vi "Periodic Tasks.vi"(8 "error in":errorcluster) -> ()   [LabVIEW 2014]
doc: "This VI runs in parallel to other tasks. It can contain as many user-defined periodic loops as you need. These can carry out PID or other sorts of timed response."
uses:
  Robot Global Data.vi
panel:
  out "Slide A 2":dbl(slide) scale=0.0..60.0
  out "Slide A":dbl(slide) scale=0.0..60.0
  out "Lift B Height":dbl format="%#_13g"
  out "Lift A Height":dbl format="%#_13g"
  in  "Reset Zero Position":bool
  out "Angle":dbl(knob) scale=0.0..360.0
  in  "stop":bool
  in  "# Items to Lift":i32=1 min=0 max=4 step=1
  out "A Up":dbl
  out "A Down":dbl
  out "B Up":dbl
  out "B Down":dbl
  out "Encoder B":dbl
  out "Encoder A":dbl
  out "Rate B":dbl
  out "Rate A":dbl
  in  "Arcade Drive?":bool
  # "Adjust the Move Lift Parameters\nto  control the speed of each lift."
  # "Tank Drive Indicators"
  # "GYRO Stuff Here"
  # "This will display the current gyro angle."
  # "The items to lift control the motor gain for raising\nand lowering in different situations.  There is a zero setting\nfor moving the motors without a tote.\n\nTo change these go to the Global Variable section and change\nthe items there (make them the default settings)."
  # "This can be set while running."
  # "Analog Devices\nADW22307"
  # "Generic Gyro Wiring:\nroboRIO AI0 S (white wire) to gyro RATE\nroboRIO AI0 V (red wire) to gyro 5V\nroboRIO AI0     (black wire) to gyro GND"
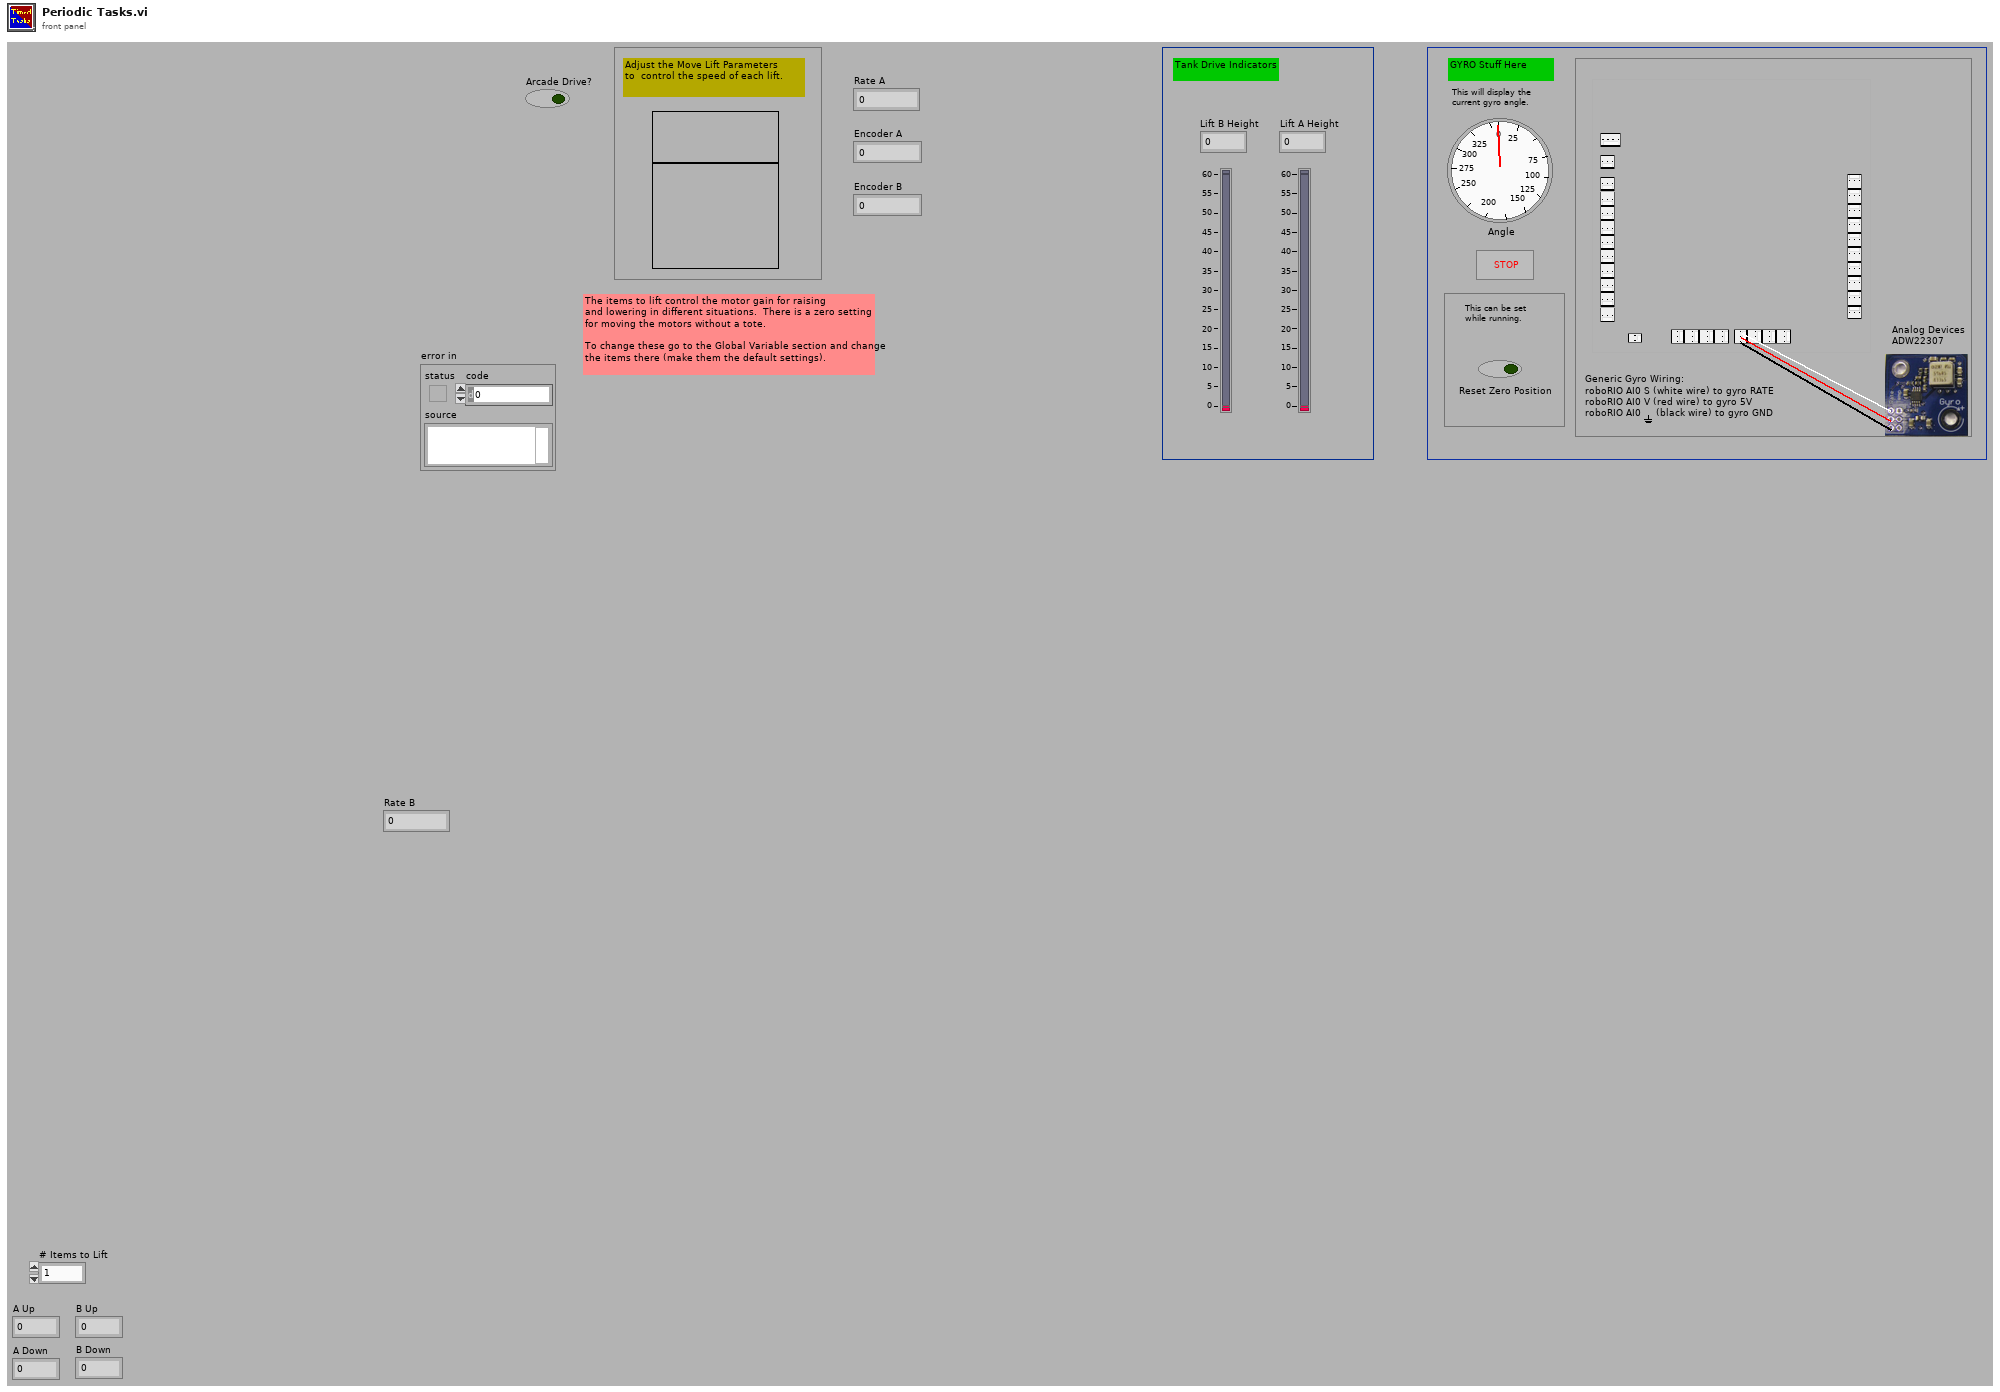
[diagram p1: front panel]
types:
  T1 = typedef "WPI_EncoderDevRef.ctl" = cluster{"DevStatus":errorcluster, "EncoderIndex":T2, "CounterIndex":T3, "DistancePerCount":dbl, "Decoding Type":T4}
  T2 = typedef "FPGA_EncoderIdx.ctl" = enum8{"Enc 0", "Enc 1", "Enc 2", "Enc 3", "Enc 4", "Enc 5", "Enc 6", "Enc 7", "Invalid"}
  T3 = typedef "FPGA_CounterCtrSystemIndex.ctl" = enum8{"Ctr 0", "Ctr 1", "Ctr 2", "Ctr 3", "Ctr 4", "Ctr 5", "Ctr 6", "Ctr 7", "Invalid"}
  T4 = typedef "WPI_EncoderType.ctl" = enum16{"1x", "2x", "4x"}
  T5 = typedef "WPI_RobotDriveDevRef.ctl" = cluster{"DevStatus":errorcluster, "Motors[]":T6[], "Square Inputs":bool, "Max Output":dbl}
  T6 = typedef "WPI_MotorControlDeviceRef.ctl" = cluster{"DeviceStatus":errorcluster, "Type":T7, "PWM":cluster{"Controller":T8, "PWM Channel":T9, "DeadBand":T10}, "CAN":cluster{"Device Number":u8, "Control Mode":T11, "Semaphore":T12, "Max Vout":dbl, "TalonSRX Control Mode":T13}, "Invert":bool, "TransformRef":T14, "InvTransformRef":T14}
  T7 = typedef "WPI_MotorControlType.ctl" = enum16{"PWM", "CAN", "CANTalonSRX"}
  T8 = typedef "FPGA_TypedefDigitalModule.ctl" = enum16{"Controller 1"}
  T9 = typedef "FPGA_DIOPWMChannel.ctl" = enum8{"PWM 0", "PWM 1", "PWM 2", "PWM 3", "PWM 4", "PWM 5", "PWM 6", "PWM 7", "PWM 8", "PWM 9", "PWM MXP 0", "PWM MXP 1", "PWM MXP 2", "PWM MXP 3", "PWM MXP 4", "PWM MXP 5", "PWM MXP 6", "PWM MXP 7", "PWM MXP 8", "PWM MXP 9", "Invalid"}
  T10 = typedef "WPI_PWMDeadband.ctl" = cluster{"Name":string, "maxPositivePwm":i32, "minPositivePwm":i32, "centerPwm":i32, "maxNegativePwm":i32, "minNegativePwm":i32, "angularRange":u16}
  T11 = typedef "WPI_CANJaguar_ControlMode.ctl" = enum8{"Percent VBus", "Current", "Speed", "Position", "Voltage"}
  T12 = typedef "Semaphore RefNum" = refnum<k1>
  T13 = typedef "WPI_CANTalonSRX_APIControlMode.ctl" = enum8{"Percent VBus", "Speed", "Position", "Slave", "Unchanged / Invalid"}
  T14 = typedef "WPI_PWMTransform_ConPane.ctl" = refnum<vi>
  T15 = typedef "WPI_JoystickDevRef.ctl" = cluster{"Device":T16}
  T16 = typedef "WPI_JoystickDeviceEnum.ctl" = enum16{"USB 0", "USB 1", "USB 2", "USB 3", "USB 4", "USB 5"}
  T17 = cluster{"Axes[0]":dbl, "Axes[1]":dbl, "Axes[2]":dbl, "Axes[3]":dbl, "Axes[4]":dbl, "Axes[5]":dbl, "Axes[6]":dbl, "Axes[7]":dbl, "Axes[8]":dbl}
  T18 = cluster{"JoystickDevRef":T15, "RobotDriveDevRef":T5}
  T19 = typedef "WPI_GyroDevRef.ctl" = cluster{"DevStatus":errorcluster, "Analog Module":T20, "Analog Channel":T21, "Offset":dbl, "Gain (VoltsPerDegree/Second)":dbl}
  T20 = typedef "FPGA_TypedefAnalogModule.ctl" = enum16{"Controller 1"}
  T21 = typedef "FPGA_AIChannel.ctl" = enum8{"AI 0", "AI 1", "AI 2", "AI 3", "AI MXP 0", "AI MXP 1", "AI MXP 2", "AI MXP 3", "Invalid"}
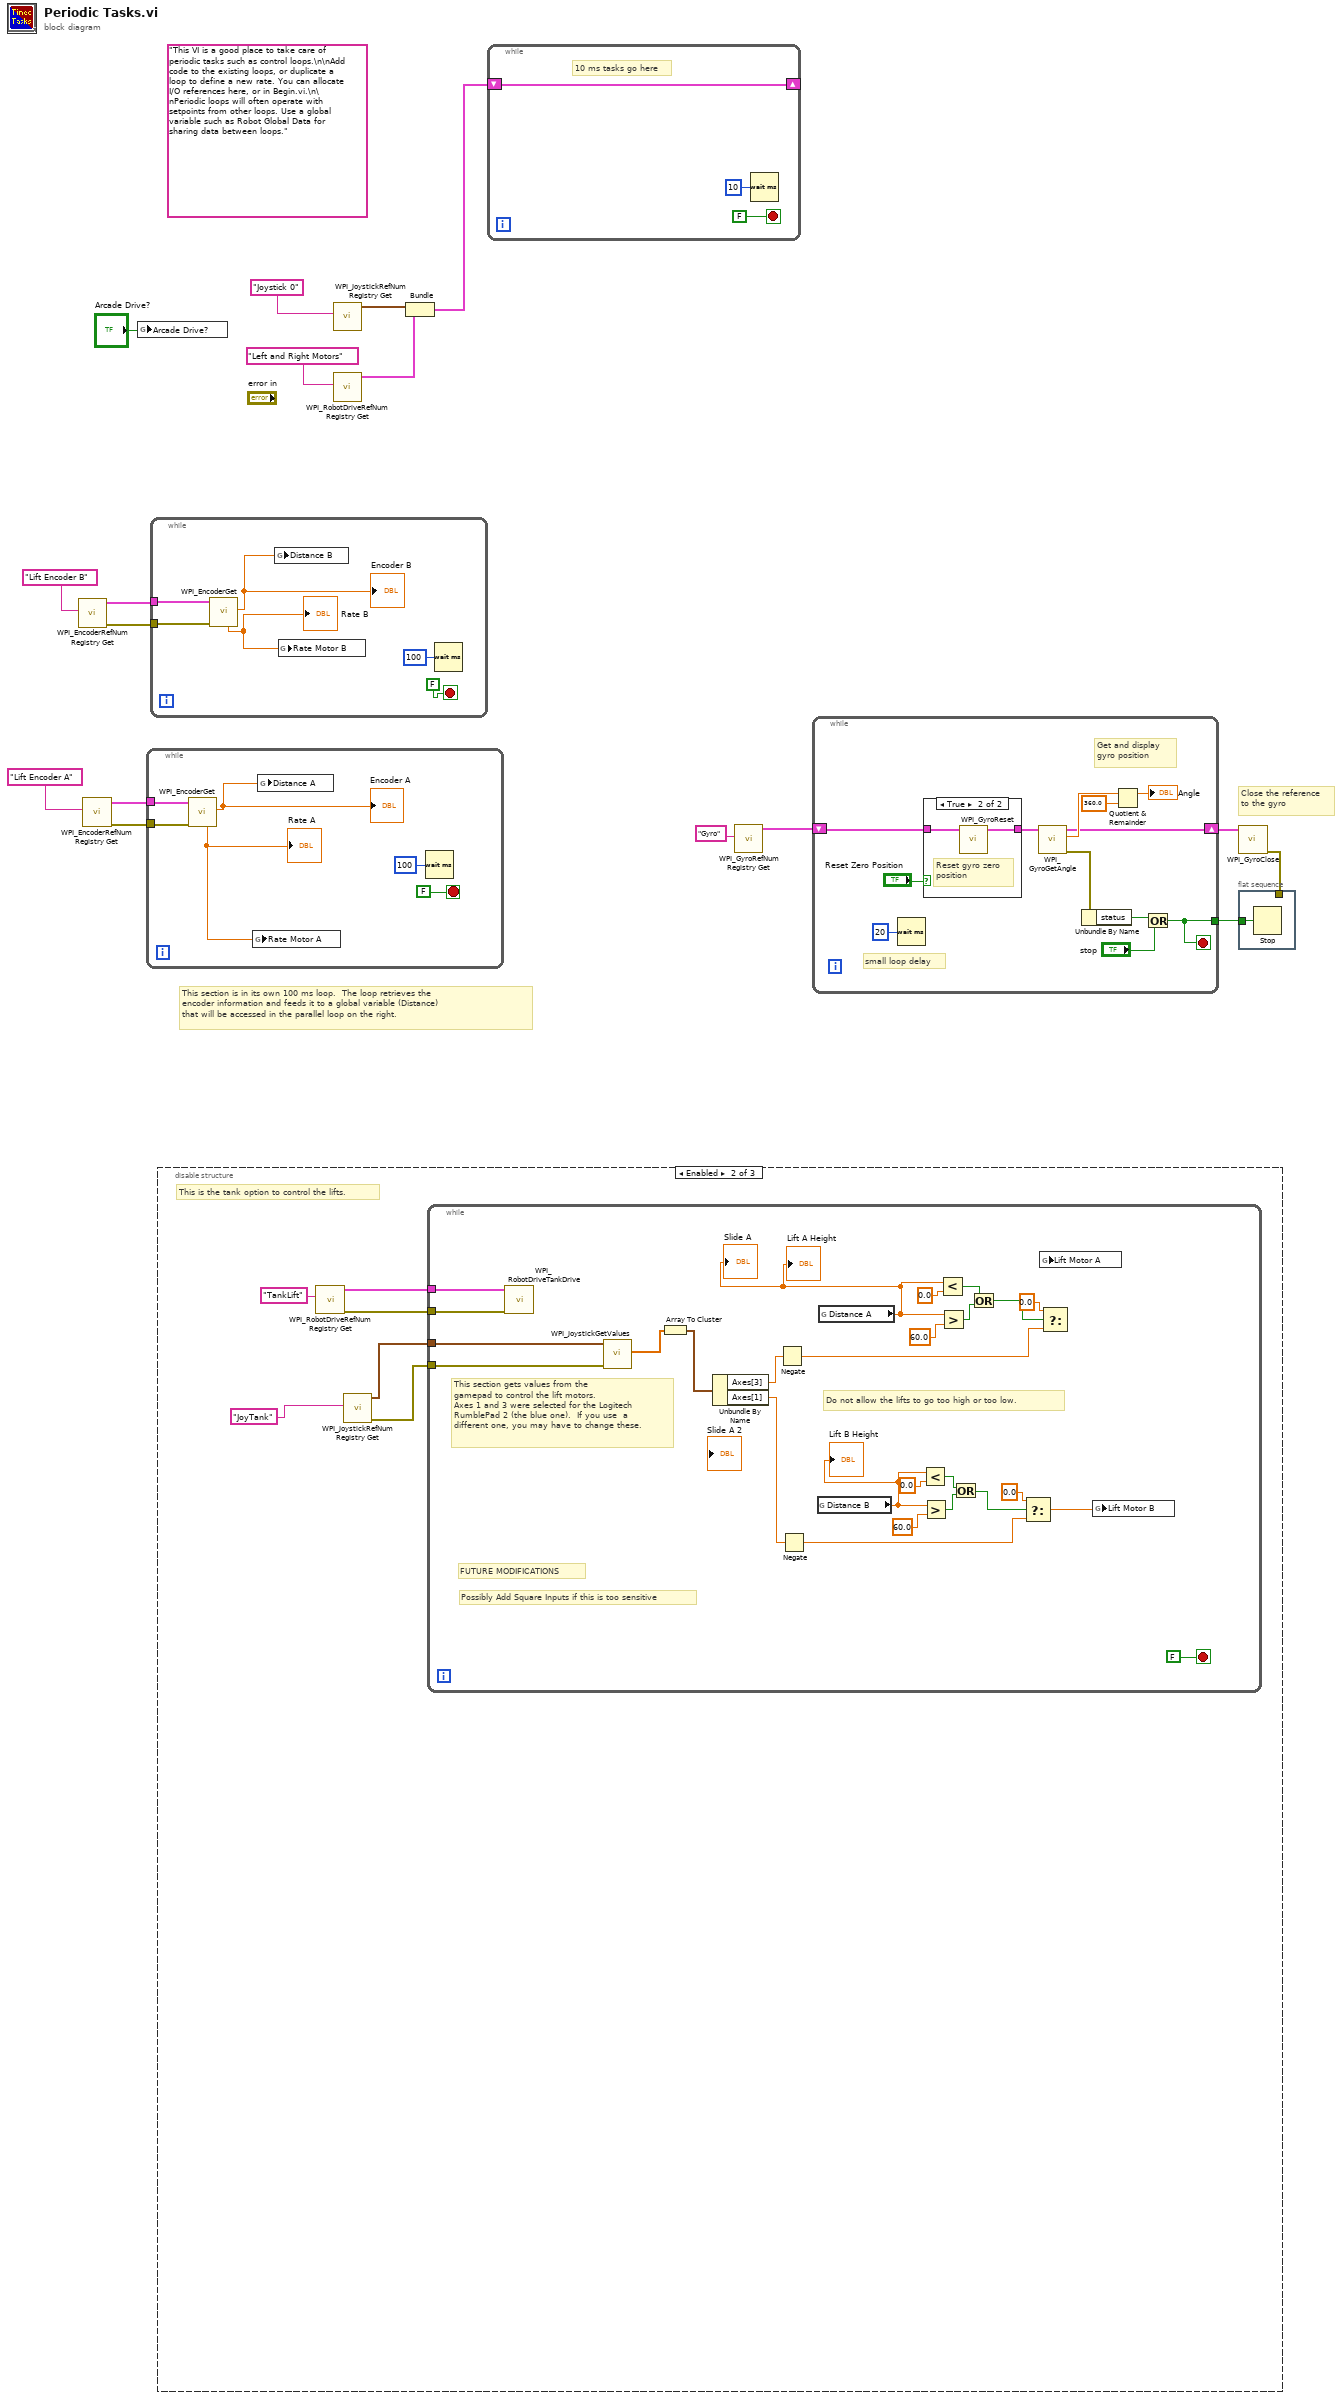
[diagram p0: block diagram]
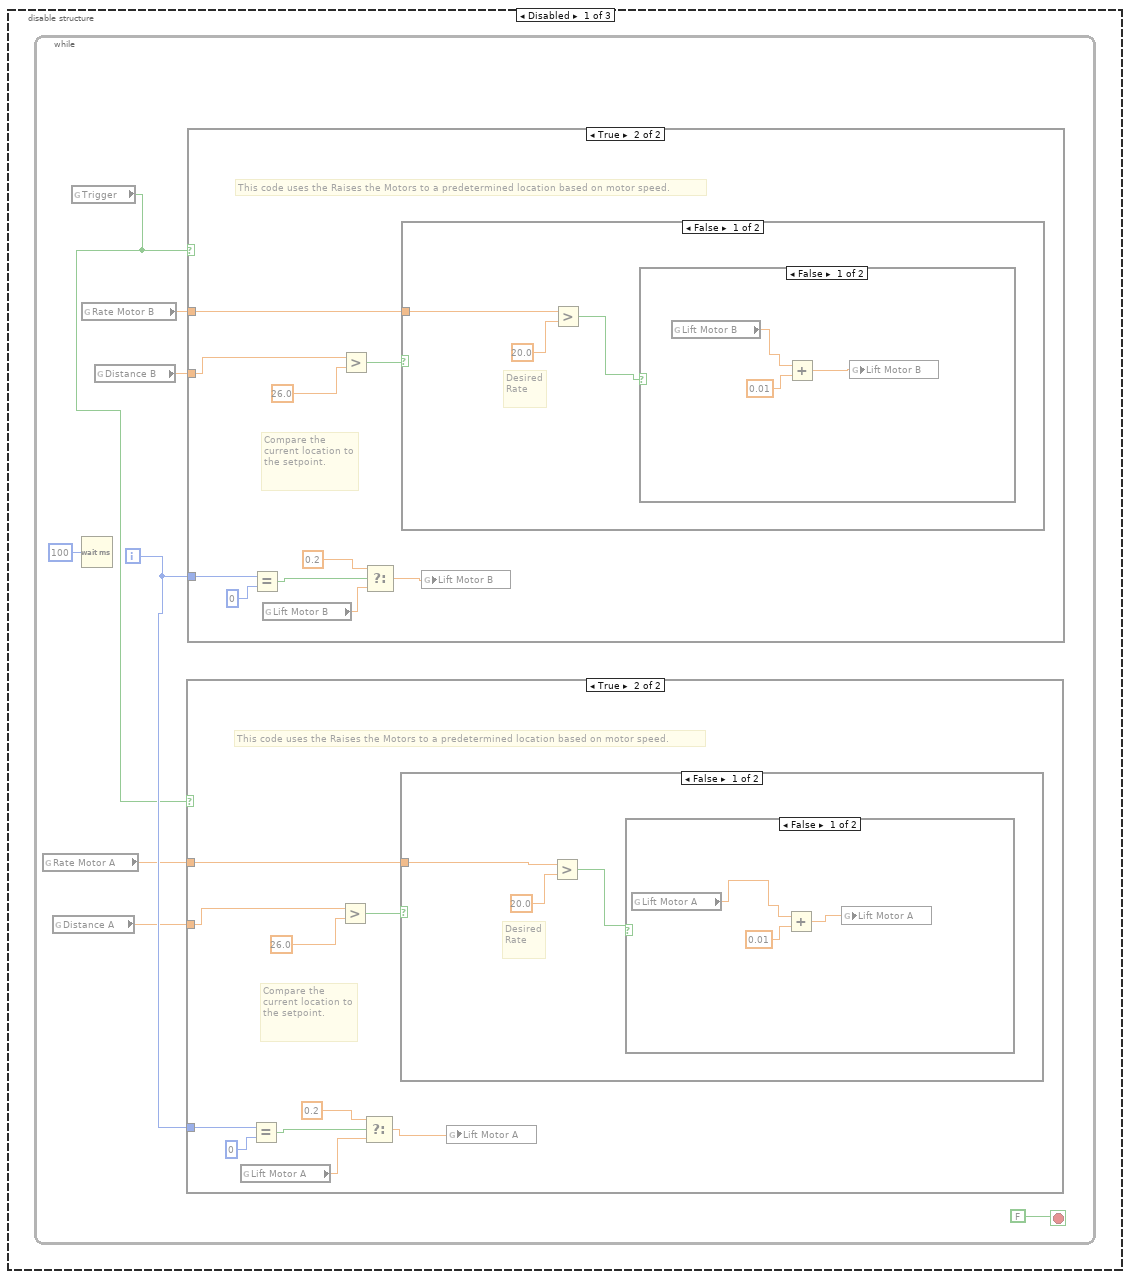
[diagram p3: hidden frame]
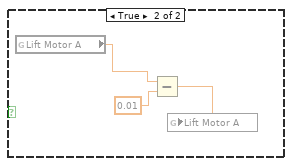
[diagram p5: hidden frame]
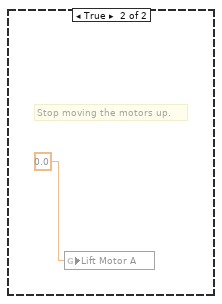
[diagram p6: hidden frame]
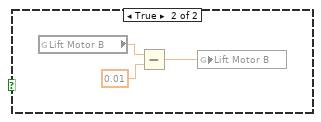
[diagram p8: hidden frame]
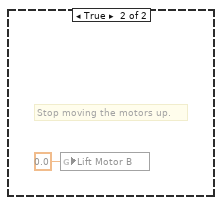
[diagram p9: hidden frame]
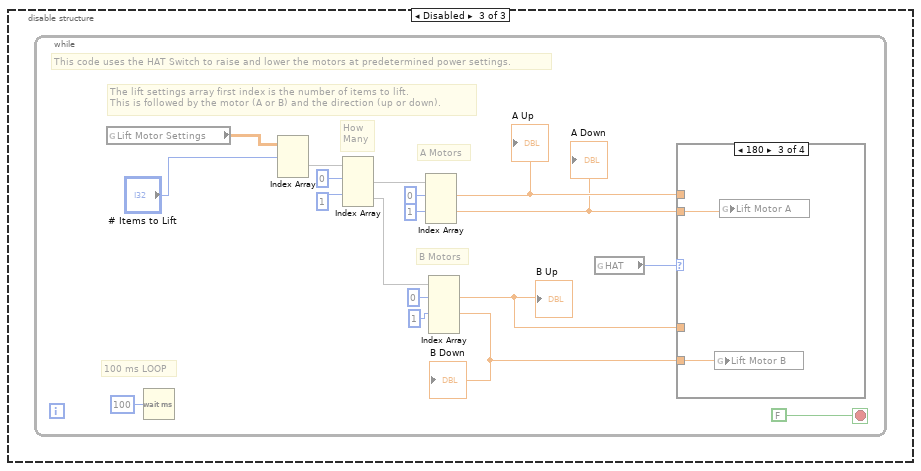
[diagram p10: hidden frame]
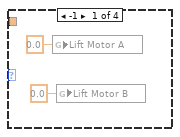
[diagram p11: hidden frame]
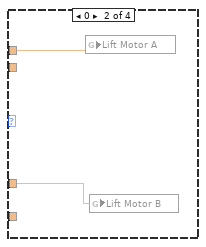
[diagram p12: hidden frame]
diagram:
  (unwired) "This VI is a good place to take care of periodic tasks such as control loops.\n\nAdd code to the existing loops, or duplicate a loop to define a new rate. You can allocate I/O references here, or in Begin.vi.\n\nPeriodic loops will often operate with setpoints from other loops. Use a global variable such as Robot Global Data for sharing data between loops."
  # "Close the reference\nto the gyro"
  # "This section is in its own 100 ms loop.  The loop retrieves the\nencoder information and feeds it to a global variable (Distance)\nthat will be accessed in the parallel loop on the right."
  n1 = call <vilib>:"WPI_EncoderRefNum Registry Get.vi"("refnum name"="Lift Encoder B") -> ("error out"=w6:errorcluster, "EncoderDevRef"=w7:T1)  [unwired: 9 in]
  n2 = call <vilib>:"WPI_EncoderRefNum Registry Get.vi"("refnum name"="Lift Encoder A") -> ("error out"=w8:errorcluster, "EncoderDevRef"=w9:T1)  [unwired: 9 in]
  n3 = global write "Robot Global Data.vi" "Arcade Drive?"("Arcade Drive?") -> ()
  n4 = while {
    tunnel: w9 -> [w21]
    tunnel: w8 -> [w20]
    stop <- FALSE stop-if-true
    n5 = call <vilib>:"WPI_EncoderGet.vi"("error in (no error)"=w20, "EncoderDevRef"=w21) -> ("Distance"=w19:dbl, "Rate"=w18:dbl)  [unwired: 4 in, 4 out]
    "Rate A" <- w18
    "Encoder A" <- w19
    n6 = global write "Robot Global Data.vi" "Rate Motor A"(w18) -> ()
    n7 = global write "Robot Global Data.vi" "Distance A"(w19) -> ()
    n8 = Wait (ms)(milliseconds to wait=u32 100) -> ()  [unwired: 1 out]
  }
  n9 = while {
    tunnel: w7 -> [w27]
    tunnel: w6 -> [w26]
    stop <- FALSE stop-if-true
    n10 = call <vilib>:"WPI_EncoderGet.vi"("error in (no error)"=w26, "EncoderDevRef"=w27) -> ("Distance"=w29:dbl, "Rate"=w28:dbl)  [unwired: 4 in, 4 out]
    "Rate B" <- w28
    "Encoder B" <- w29
    n11 = global write "Robot Global Data.vi" "Distance B"(w29) -> ()
    n12 = global write "Robot Global Data.vi" "Rate Motor B"(w28) -> ()
    n13 = Wait (ms)(milliseconds to wait=u32 100) -> ()  [unwired: 1 out]
  }
  n14 = disable-structure shown="Enabled" {
    frame Disabled {
      n15 = while {
        i -> [w33]
        stop <- FALSE stop-if-true
        n16 = global read "Robot Global Data.vi" "Rate Motor A"() -> (w31:dbl)
        n17 = global read "Robot Global Data.vi" "Distance A"() -> (w30:dbl)
        n18 = global read "Robot Global Data.vi" "Trigger"() -> (w32:bool)
        n19 = global read "Robot Global Data.vi" "Rate Motor B"() -> (w34:dbl)
        n20 = Wait (ms)(milliseconds to wait=u32 100) -> ()  [unwired: 1 out]
        n21 = global read "Robot Global Data.vi" "Distance B"() -> (w35:dbl)
        n22 = case shown="True" w32 {
          tunnel: w30 -> [_ w44]
          tunnel: w31 -> [_ w46]
          tunnel: w33 -> [_ w43]
          frame False {
          }
          frame True {
            # "Compare the current location to the setpoint."
            # "This code uses the Raises the Motors to a predetermined location based on motor speed."
            n23 = global read "Robot Global Data.vi" "Lift Motor A"() -> (w38:dbl)
            n24 = Equal?(x=w43, y=0) -> (x = y?=w41:bool)
            n25 = Greater?(x=w44, y=26.0 ("x")) -> (0:w47:bool)
            n26 = Select(t=0.2, s=w41, f=w38) -> (s? t:f=w39:dbl)
            n27 = case shown="False" w47 {
              tunnel: w46 -> [w48 _]
              frame False {
                # "Desired\nRate"
                n28 = Greater?(x=w48, y=20.0 ("x")) -> (0:w50:bool)
                n29 = case shown="False" w50 {
                  frame False {
                    n30 = global read "Robot Global Data.vi" "Lift Motor A"() -> (w51:dbl)
                    n31 = Add(x=w51, y=0.01) -> (x+y=w52:dbl)
                    n32 = global write "Robot Global Data.vi" "Lift Motor A"(w52) -> ()
                  }
                  frame True {
                    n33 = global read "Robot Global Data.vi" "Lift Motor A"() -> (w54:dbl)
                    n34 = Subtract(x=w54, y=0.01) -> (x-y=w55:dbl)
                    n35 = global write "Robot Global Data.vi" "Lift Motor A"(w55) -> ()
                  }
                }
              }
              frame True {
                # "Stop moving the motors up."
                n36 = global write "Robot Global Data.vi" "Lift Motor A"(0.0 ("Lift Motor B")) -> ()
              }
            }
            n37 = global write "Robot Global Data.vi" "Lift Motor A"(w39) -> ()
          }
        }
        n38 = case shown="True" w32 {
          tunnel: w35 -> [_ w64]
          tunnel: w34 -> [_ w66]
          tunnel: w33 -> [_ w63]
          frame False {
          }
          frame True {
            # "Compare the current location to the setpoint."
            # "This code uses the Raises the Motors to a predetermined location based on motor speed."
            n39 = Equal?(x=w63, y=0) -> (x = y?=w61:bool)
            n40 = global read "Robot Global Data.vi" "Lift Motor B"() -> (w58:dbl)
            n41 = Greater?(x=w64, y=26.0 ("x")) -> (0:w67:bool)
            n42 = Select(t=0.2, s=w61, f=w58) -> (s? t:f=w59:dbl)
            n43 = case shown="False" w67 {
              tunnel: w66 -> [w68 _]
              frame False {
                # "Desired\nRate"
                n44 = Greater?(x=w68, y=20.0 ("x")) -> (0:w70:bool)
                n45 = case shown="False" w70 {
                  frame False {
                    n46 = global read "Robot Global Data.vi" "Lift Motor B"() -> (w71:dbl)
                    n47 = Add(x=w71, y=0.01) -> (x+y=w72:dbl)
                    n48 = global write "Robot Global Data.vi" "Lift Motor B"(w72) -> ()
                  }
                  frame True {
                    n49 = global read "Robot Global Data.vi" "Lift Motor B"() -> (w76:dbl)
                    n50 = Subtract(x=w76, y=0.01) -> (x-y=w74:dbl)
                    n51 = global write "Robot Global Data.vi" "Lift Motor B"(w74) -> ()
                  }
                }
              }
              frame True {
                # "Stop moving the motors up."
                n52 = global write "Robot Global Data.vi" "Lift Motor B"(0.0 ("Lift Motor B")) -> ()
              }
            }
            n53 = global write "Robot Global Data.vi" "Lift Motor B"(w59) -> ()
          }
        }
      }
    }
    frame Enabled {
      # "This is the tank option to control the lifts."
      n54 = call <vilib>:"WPI_RobotDriveRefNum Registry Get.vi"("refnum name"="TankLift") -> ("error out"=w81:errorcluster, "RobotDriveDevRef"=w82:T5)  [unwired: 9 in]
      n55 = call <vilib>:"WPI_JoystickRefNum Registry Get.vi"("refnum name"="JoyTank") -> ("error out"=w78:errorcluster, "JoystickDevRef"=w79:T15)  [unwired: 9 in]
      n56 = while {
        tunnel: w82 -> [w109]
        tunnel: w81 -> [w108]
        tunnel: w79 -> [w102]
        tunnel: w78 -> [w101]
        stop <- FALSE stop-if-true
        # "Possibly Add Square Inputs if this is too sensitive"
        # "Do not allow the lifts to go too high or too low."
        # "FUTURE MODIFICATIONS"
        # "This section gets values from the \ngamepad to control the lift motors.\nAxes 1 and 3 were selected for the Logitech\nRumblePad 2 (the blue one).  If you use  a\ndifferent one, you may have to change these."
        n57 = call <vilib>:"WPI_RobotDriveTankDrive.vi"("error in (no error)"=w108, "RobotDriveDevRef"=w109) -> ()  [unwired: 7 in, 3 out]
        n58 = call <vilib>:"WPI_JoystickGetValues.vi"("error in (no error)"=w101, "JoystickDevRef"=w102) -> ("Axes"=w105:dbl[])  [unwired: 5 in, 4 out]
        n59 = Array To Cluster(array=w105) -> (cluster=w106:T17)
        n60 = Unbundle By Name(w106) -> ("Axes[3]"=w104:dbl, "Axes[1]"=w103:dbl)
        n61 = Negate(x=w104) -> (-x=w86:dbl)
        n62 = Negate(x=w103) -> (-x=w98:dbl)
        n63 = global read "Robot Global Data.vi" "Distance B"() -> (w85:dbl)
        "Lift B Height" <- w85
        n64 = global read "Robot Global Data.vi" "Distance A"() -> (w84:dbl)
        "Lift A Height" <- w84
        "Slide A" <- w84
        n65 = Less?(x=w85, y=0.0) -> (x < y?=w95:bool)
        n66 = Greater?(x=w85, y=60.0) -> (0:w96:bool)
        n67 = Less?(x=w84, y=0.0) -> (x < y?=w88:bool)
        n68 = Greater?(x=w84, y=60.0) -> (0:w89:bool)
        n69 = Or(x=w95, y=w96) -> (x .or. y?=w94:bool)
        n70 = Or(x=w88, y=w89) -> (x .or. y?=w87:bool)
        n71 = Select(t=0.0, s=w94, f=w98) -> (s? t:f=w93:dbl)
        n72 = global read "Robot Global Data.vi" "Lift Motor A"() -> ()  [unwired: 1 in]
        n73 = Select(t=0.0, s=w87, f=w86) -> ()  [unwired: 1 out]
        n74 = global write "Robot Global Data.vi" "Lift Motor B"(w93) -> ()
      }
    }
    frame Disabled {
      n75 = while {
        stop <- FALSE stop-if-true
        # "B Motors"
        # "A Motors"
        # "How\nMany"
        # "The lift settings array first index is the number of items to lift.\nThis is followed by the motor (A or B) and the direction (up or down)."
        # "This code uses the HAT Switch to raise and lower the motors at predetermined power settings."
        # "100 ms LOOP"
        n76 = global read "Robot Global Data.vi" "Lift Motor Settings"() -> (w124:dbl[][][])
        n77 = Wait (ms)(milliseconds to wait=u32 100) -> ()  [unwired: 1 out]
        n78 = Index Array(array=w124, index (dim 0)="# Items to Lift") -> (element=w123:dbl[][])  [unwired: 2 in]
        n79 = Index Array(array=w123, index (row) #1=0 ("index (row)"), index (row) #2=1 ("index (row)")) -> (element #1=w120:dbl[], element #2=w119:dbl[])  [unwired: 2 in]
        n80 = Index Array(array=w120, index #1=0 ("index"), index #3=1 ("index")) -> (element #1=w114:dbl, element #3=w113:dbl)  [unwired: 2 in, 2 out]
        "A Up" <- w114
        "A Down" <- w113
        n81 = Index Array(array=w119, index #1=0 ("index"), index #3=1 ("index")) -> (element #1=w111:dbl, element #3=w112:dbl)  [unwired: 3 in, 3 out]
        "B Up" <- w111
        "B Down" <- w112
        n82 = global read "Robot Global Data.vi" "HAT"() -> (w125:i16)
        n83 = case shown="180" w125 {
          tunnel: w114 -> [_ w131 _ _]
          tunnel: w113 -> [_ _ w133 _]
          tunnel: w112 -> [_ _ w132 _]
          tunnel: w111 -> [_ w130 _ _]
          frame -1 {
            n84 = global write "Robot Global Data.vi" "Lift Motor A"(0.0 ("Lift Motor A")) -> ()
            n85 = global write "Robot Global Data.vi" "Lift Motor B"(0.0 ("Lift Motor A")) -> ()
          }
          frame 0 {
            n86 = global write "Robot Global Data.vi" "Lift Motor A"(w131) -> ()
            n87 = global write "Robot Global Data.vi" "Lift Motor B"(w130) -> ()
          }
          frame 180 {
            n88 = global write "Robot Global Data.vi" "Lift Motor B"(w132) -> ()
            n89 = global write "Robot Global Data.vi" "Lift Motor A"(w133) -> ()
          }
          frame Default {
          }
        }
      }
    }
  }
  n90 = call <vilib>:"WPI_JoystickRefNum Registry Get.vi"("refnum name"="Joystick 0") -> ("JoystickDevRef"=w15:T15)  [unwired: 1 in, 9 out]
  n91 = call <vilib>:"WPI_RobotDriveRefNum Registry Get.vi"("refnum name"="Left and Right Motors") -> ("RobotDriveDevRef"=w14:T5)  [unwired: 1 in, 9 out]
  n92 = Bundle("JoystickDevRef"=w15, "RobotDriveDevRef"=w14) -> (w13:T18)  [unwired: 1 out]
  n93 = while {
    shift-right: [w134] -> _
    shift-left: w13 -> [w134]
    stop <- FALSE stop-if-true
    # "10 ms tasks go here"
    n94 = Wait (ms)(milliseconds to wait=u32 10) -> ()  [unwired: 1 out]
  }
  n95 = call <vilib>:"WPI_GyroRefNum Registry Get.vi"("refnum name"="Gyro") -> ("GyroDevRef"=w1:T19)  [unwired: 9 in, 1 out]
  n96 = while {
    shift-right: [w144] -> w5
    shift-left: w1 -> [w147]
    tunnel: [w142] -> w4
    stop <- w142 stop-if-true
    # "small loop delay"
    # "Get and display\ngyro position"
    n97 = Wait (ms)(milliseconds to wait=u32 20) -> ()  [unwired: 1 out]
    n98 = case shown="True" "Reset Zero Position" {
      tunnel: w147 -> [w149 w151]
      tunnel: [w149 w150] -> w146
      frame False {
      }
      frame True {
        # "Reset gyro zero \nposition"
        n99 = call <vilib>:"WPI_GyroReset.vi"("GyroDevRef"=w151) -> ("GyroDevRef"=w150:T19)  [unwired: 10 out]
      }
    }
    n100 = call <vilib>:"WPI_GyroGetAngle.vi"("GyroDevRef"=w146) -> ("error out"=w138:errorcluster, "Angle"=w145:dbl, "GyroDevRef"=w144:T19)  [unwired: 1 in, 7 out]
    n101 = Unbundle By Name(w138) -> ("status"=w143:bool)
    n102 = Quotient & Remainder(x=w145, y=360.0) -> (x-y*floor(x/y)=→"Angle":dbl)  [unwired: 1 out]
    n103 = Or(x=w143, y="stop") -> (x .or. y?=w142:bool)
  }
  n104 = call <vilib>:"WPI_GyroClose.vi"("GyroDevRef"=w5) -> ("error out"=w3:errorcluster)  [unwired: 1 in, 9 out]
  n105 = flat-sequence {
    tunnel: w4 -> [w152]
    tunnel: w3 -> [_]
    frame #0 {
      n106 = Stop(stop? (T)=w152) -> ()
    }
  }
